vi "VI-Get Icon As Template.vi"(0 "VIref in":refnum<vi>, 7 "Prefix":string, 11 "error in (no error)":errorcluster) -> (4 "VIref out":refnum<vi>, 10 "Icon Framework.lvclass out":refnum<class "Icon Framework.lvclass">, 15 "error out":errorcluster)   [LabVIEW 2020]
uses:
  <vilib>/LabVIEW Icon API/lv_icon/Classes/Icon Framework/Icon Framework.lvclass
  <vilib>/LabVIEW Icon API/lv_icon/Controls/Pathes.ctl
  <vilib>/LabVIEW Icon API/LabVIEW Icon API.lvlib
  <vilib>/LabVIEW Icon API/lv_icon/lv_icon.lvlib
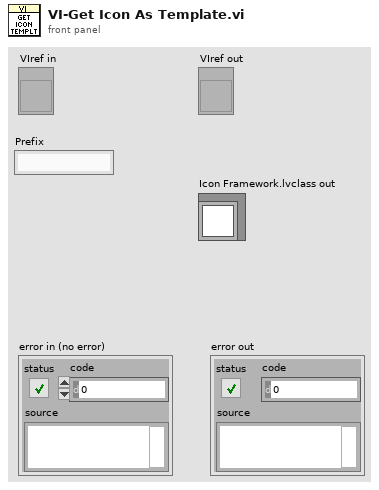
[diagram p1: front panel]
types:
  T1 = typedef "Pathes.ctl" = enum16{"Root Path", "Icon Templates", "Icon Templates VI", "Icon Templates Lib", "Glyphs"}
  T2 = typedef "imagedata.ctl" = cluster{"image type":i32, "image depth":i32, "image":u8[], "mask":u8[], "colors":u32[], "Rectangle":cluster{"left":i16, "top":i16, "right":i16, "bottom":i16}}
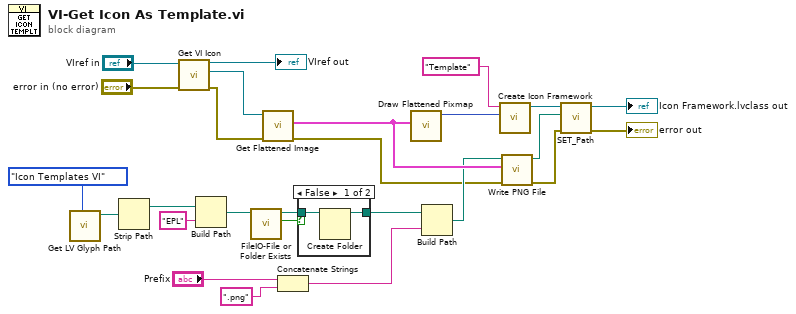
[diagram p0: block diagram]
diagram:
  n1 = call <vilib>:"Get LV Glyph Path.vi"("Path"=Pathes."Icon Templates VI") -> ("Requested Path"=w11:path)  [unwired: 2 in, 8 out]
  n2 = Strip Path(path=w11) -> (stripped path=w10:path)  [unwired: 1 out]
  n3 = call <vilib>:"Get VI Icon.vi"("error in (no error)"="error in (no error)", "VI Refnum in"="VIref in") -> ("error out"=w23:errorcluster, "Icon"=w24:refnum<class "Icon.lvclass">, "VI Refnum out"=→"VIref out":refnum<vi>)  [unwired: 7 in]
  n4 = Build Path(base path=w10, name or relative path="EPL") -> (appended path=w9:path)
  n5 = call "FileIO-File or Folder Exists.vi"("path"=w9) -> ("Directory?"=w8:bool, "dup path"=w7:path)  [unwired: 7 in, 2 out]
  n6 = call <vilib>:"Get Flattened Image.vi"("error in (no error)"=w23, "lv_icon.lvlib:Icon.lvclass in"=w24) -> ("error out"=w2:errorcluster, "Color Image"=w14:T2)  [unwired: 6 in, 2 out]
  n7 = Concatenate Strings("Prefix", ".png" ("string")) -> (w5:string)
  n8 = case shown="False" w8 {
    tunnel: w7 -> [w28 w29]
    tunnel: [w27 w29] -> w6
    frame False {
      n9 = Create Folder(path (use dialog)=w28) -> (created path=w27:path)  [unwired: 2 in, 2 out]
    }
    frame True {
    }
  }
  n10 = call <vilib>:"Draw Flattened Pixmap.vi"("image data"=w14) -> ("new picture"=w20:picture)  [unwired: 8 in]
  n11 = Build Path(base path=w6, name or relative path=w5) -> (appended path=w13:path)
  n12 = call <vilib>:"Create Icon Framework.vi"("Template Glyph"=w20, "Layer name"="Template" ("Template Layer")) -> ("Icon Framework out"=w21:refnum<class "Icon Framework.lvclass">)  [unwired: 9 in]
  n13 = call <vilib>:"Write PNG File.vi"("error in (no error)"=w2, "image data"=w14, "path to PNG file"=w13) -> ("error out"=w3:errorcluster, "path"=w12:path)  [unwired: 7 in]
  n14 = call <vilib>:"SET_Path.vi"("error in (no error)"=w3, "Path"=w12, "Icon Framework.lvclass in"=w21) -> ("error out"=→"error out":errorcluster, "Icon Framework.lvclass out"=→"Icon Framework.lvclass out":refnum<class "Icon Framework.lvclass">)  [unwired: 7 in]
